vi "Get-FP-All-Ctrl-Ref.vi"(8 "error in (no error)":errorcluster, 11 "VI Refnum":refnum<vi>) -> (0 "error out":errorcluster, 3 "Quick-GUI-Update out":refnum<class "Quick-GUI-Update.lvclass">)   [LabVIEW 2020, in "Quick-GUI-Update.lvclass"]
uses:
  Quick-GUI-Update.lvclass
  Ctrl Reference's/Ctrl Reference's.lvclass
  Quick-GUI-Update.lvclass/Quick-GUI-Update.ctl
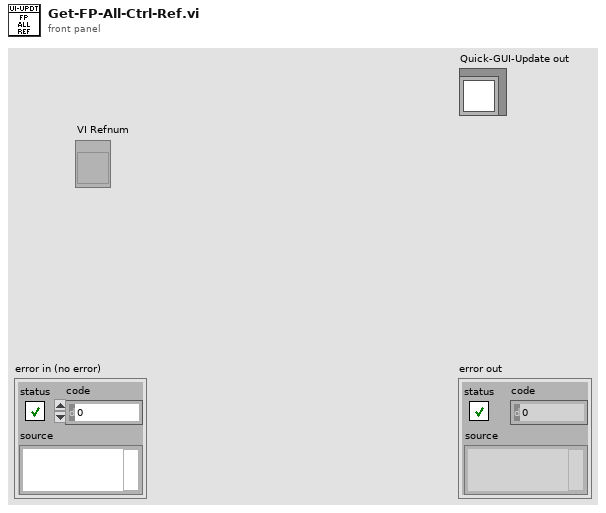
[diagram p1: front panel]
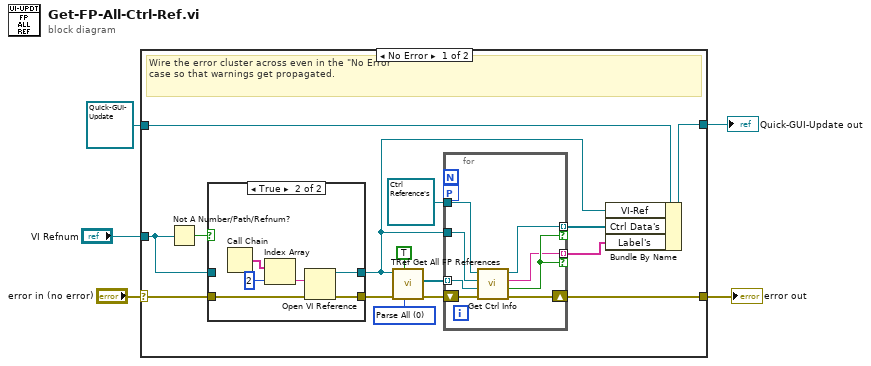
[diagram p0: block diagram]
diagram:
  n1 = case shown="No Error" "error in (no error)" {
    selector: "error in (no error)" -> [w14 w38]
    tunnel: [w15 w38] -> w4
    tunnel: [w19 w37] -> w2
    tunnel: refnum<class "Quick-GUI-Update.lvclass"> refnum ("Quick-GUI-Update in") -> [w20 w37]
    tunnel: "VI Refnum" -> [w13 _]
    frame No Error {
      w10 = u16 0 items=["Parse All", "Parse Tabs Only"] ("Parsing Rule")
      # "Wire the error cluster across even in the \"No Error\"\ncase so that warnings get propagated."
      n2 = Not A Number/Path/Refnum?(number/path/refnum=w13) -> (NaN/Path/Refnum?=w18:bool)
      n3 = case shown="True" w18 {
        tunnel: w13 -> [w30 _]
        tunnel: [w30 w31] -> w6
        tunnel: w14 -> [w29 w33]
        tunnel: [w29 w32] -> w12
        frame False {
        }
        frame True {
          n4 = Call Chain() -> (call chain=w36:string[])
          n5 = Index Array(array=w36, index=2 ("Index")) -> (element=w35:string)
          n6 = Open VI Reference(vi path=w35, error in (no error)=w33) -> (vi reference=w31:refnum<vi>, error out=w32:errorcluster)  [unwired: 4 in]
        }
      }
      n7 = call <vilib>:"TRef Get All FP References.vi"("Parsing Rule"=w10, "Ignore Decorations?"=TRUE, "error in (no error)"=w12, "VI Refnum"=w6) -> ("error out"=w16:errorcluster, "All FP Objects"=w17:refnum<vi>[])  [unwired: 3 in, 3 out]
      n8 = for {
        tunnel: w17 -> [w28] mode=indexing
        shift-right: [w23] -> w15
        shift-left: w16 -> [w24]
        tunnel: [w25] -> w9 mode=indexing if=w26
        workers-P: _ -> [_]
        tunnel: [w27] -> w8 mode=indexing if=w26
        tunnel: refnum<class "Ctrl Reference's.lvclass"> refnum ("Ctrl Reference's.lvclass") -> [w22]
        tunnel: w6 -> [w21]
        n9 = call "Get Ctrl Info.vi"("error in (no error)"=w24, "GObj Refnum"=w28, "VI-Ref"=w21, "Ctrl Reference's in"=w22) -> ("error out"=w23:errorcluster, "Has Label?"=w26:bool, "Label"=w25:string, "Ctrl Reference's out"=w27:refnum<class "Ctrl Reference's.lvclass">)  [unwired: 4 in]
      }
      n10 = Bundle By Name(cluster=w20, "VI-Ref"=w6, "Ctrl Data's"=w8, "Label's"=w9) -> (w19:refnum<class "Quick-GUI-Update.lvclass">)
    }
    frame Error {
    }
  }
  "error out" <- w4
  "Quick-GUI-Update out" <- w2
